vi "sub_vi_saving_string_calibration.vi"(0 "Received data":string[](array[string]), 1 "calculated noise":dbl, 2 "Absolute errors array":dbl[](array[numeric]), 3 "Relative errors array":dbl[](array[numeric]), 4 "calculated slope":dbl, 5 "calculated intercept":dbl, 10 "gain":dbl) -> (16 "Resulting array":string[](array[string]))   [LabVIEW 2016]
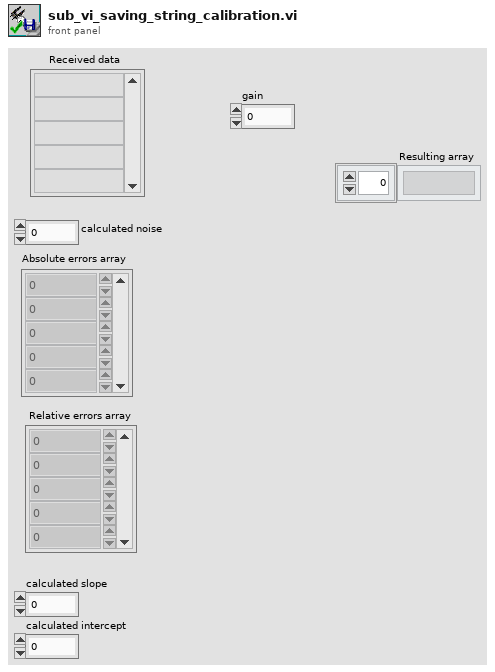
[diagram p1: front panel]
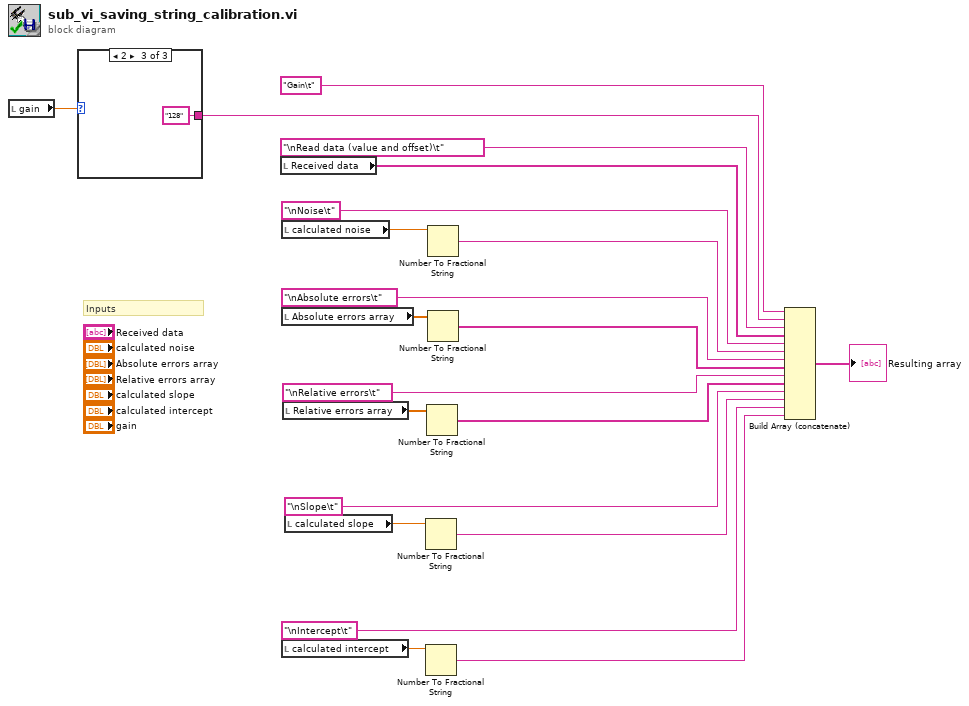
[diagram p0: block diagram]
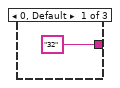
[diagram p2: hidden frame]
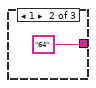
[diagram p3: hidden frame]
diagram:
  # "Inputs"
  n1 = local read "gain"() -> (w2:dbl)
  n2 = case shown="2" w2 {
    tunnel: ["32" "64" "128"] -> w1
    frame 0, Default {
    }
    frame 1 {
    }
    frame 2 {
    }
  }
  n3 = local read "Received data"() -> (w15:string[])
  n4 = local read "calculated noise"() -> (w21:dbl)
  n5 = local read "Absolute errors array"() -> (w20:dbl[])
  n6 = local read "calculated intercept"() -> (w17:dbl)
  n7 = local read "Relative errors array"() -> (w19:dbl[])
  n8 = local read "calculated slope"() -> (w18:dbl)
  n9 = Number To Fractional String(number=w18) -> (F-format string=w7:string)  [unwired: 3 in]
  n10 = Number To Fractional String(number=w17) -> (F-format string=w5:string)  [unwired: 3 in]
  n11 = Number To Fractional String(number=w19) -> (F-format string=w9:string[])  [unwired: 3 in]
  n12 = Number To Fractional String(number=w21) -> (F-format string=w13:string)  [unwired: 3 in]
  n13 = Number To Fractional String(number=w20) -> (F-format string=w11:string[])  [unwired: 3 in]
  n14 = Build Array (concatenate)("Gain\t", w1, "\nRead data (value and offset)\t", w15, "\nNoise\t", w13, "\nAbsolute errors\t", w11, "\nRelative errors\t", w9, "\nSlope\t" ("string"), w7, "\nIntercept\t" ("string"), w5) -> (→"Resulting array":string[])
